vi "wrap_JointPositions.vi"(3 "Mode":T1=1 items=["Position"=1, "Velocity"=2, "Effort"=3], 4 "Positions":dbl[](array[numeric]), 5 "Side":T2, 6 "msg in":string) -> (2 "msg out":string)   [LabVIEW 2015]
uses:
  Code/SubVIs/BaxterSide.ctl
  Code/SubVIs/JointMode.ctl
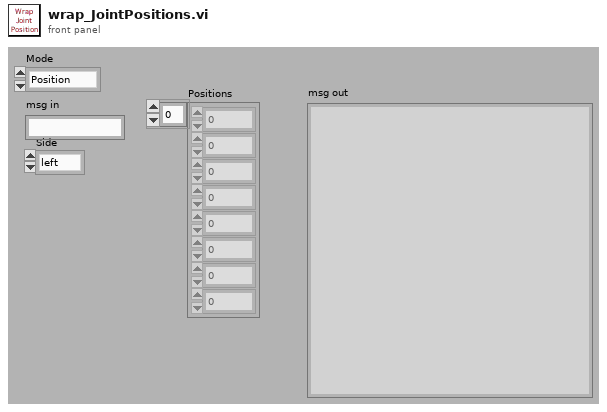
[diagram p1: front panel]
types:
  T1 = typedef "JointMode.ctl" = u8
  T2 = typedef "BaxterSide.ctl" = enum16{"left", "right"}
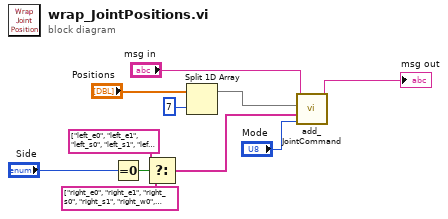
[diagram p0: block diagram]
diagram:
  n1 = Equal To 0?(x="Side") -> (x = 0?=w11:bool)
  n2 = Select(t=string[] ["left_e0", "left_e1", "left_s0", "left_s1", "left_w0", "left_w1", "left_w2"] ("left"), s=w11, f=string[] ["right_e0", "right_e1", "right_s0", "right_s1", "right_w0", "right_w1", "right_w2"] ("right")) -> (s? t:f=w2:string[])
  n3 = Split 1D Array(array="Positions", index=7) -> (first subarray=w3:dbl[])  [unwired: 1 out]
  n4 = call "add_JointCommand.vi"("Mode"="Mode", "names"=w2, "command"=w3, "msg in"="msg in") -> ("msg out"=→"msg out":string)  [unwired: 7 in]
